vi "serial_RS232.vi"() -> ()   [LabVIEW 2012]
uses:
  <vilib>/Instr/_visa.llb/VISA Configure Serial Port (Instr).vi
panel:
  in  "stop":bool
  out "read buffer":string
  in  "write buffer":string
  in  "VISA resource name":refnum<visa-resource-name>
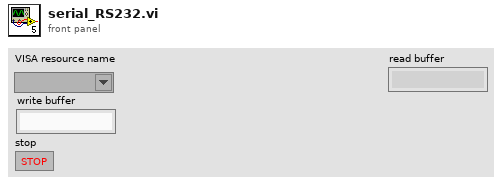
[diagram p1: front panel]
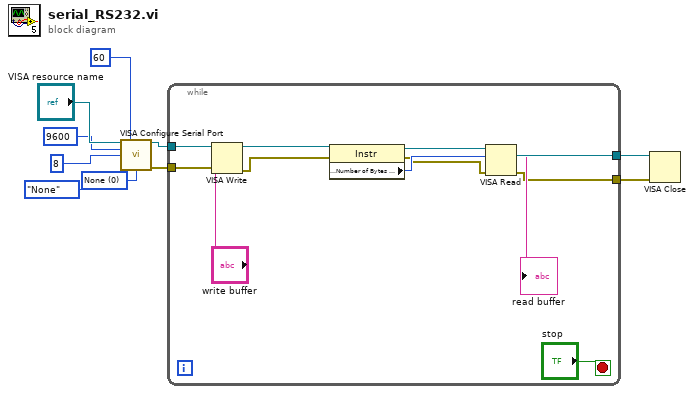
[diagram p0: block diagram]
diagram:
  w4 = u16 0 items=["None", "XON/XOFF", "RTS/CTS", "XON/XOFF & RTS/CTS", "DTR/DSR", "XON/XOFF & DTR/DSR"] ("flow control (0:none)")
  n1 = call-poly "VISA Configure Serial Port"("VISA resource name"="VISA resource name", "timeout (10sec)"=u32 60, "baud rate (9600)"=u32 9600, "data bits (8)"=u16 8, "parity (0:none)"=enum16{"None", "Odd", "Even", "Mark", "Space"}."None", "flow control (0:none)"=w4) -> ("VISA resource name out"=w10:refnum<visa-resource-name>, "error out"=w2:errorcluster)  [unwired: 8 in]
  n2 = while {
    tunnel: w10 -> [w22]
    tunnel: [w19] -> w9
    tunnel: w2 -> [w15]
    tunnel: [w12] -> w1
    stop <- "stop" stop-if-true
    n3 = VISA Write(VISA resource name=w22, write buffer="write buffer", error in (no error)=w15) -> (VISA resource name out=w21:refnum<visa-resource-name>, error out=w14:errorcluster)  [unwired: 1 out]
    n4 = property class="Instr"(reference=w21, error in=w14) -> (reference out=w20:refnum<visa-resource-name>, error out=w13:errorcluster, "Serial Settings:Number of Bytes at Serial Port"=w16:u32)
    n5 = VISA Read(VISA resource name=w20, byte count=w16, error in (no error)=w13) -> (VISA resource name out=w19:refnum<visa-resource-name>, read buffer=→"read buffer":string, error out=w12:errorcluster)  [unwired: 1 out]
  }
  n6 = VISA Close(VISA resource name=w9, error in (no error)=w1) -> ()  [unwired: 1 out]
